vi "Speed Sensitivity.vi"(10 "Joystick \nValue":dbl format="%#_13g") -> (2 "Speed\nOutput":dbl)   [LabVIEW 2014]
panel:
  in  "Shift the\nParabola":dbl
  in  "Full Power\nSetpoint":dbl=0.99 format="%#_13g"
  # "Parabolic Controls"
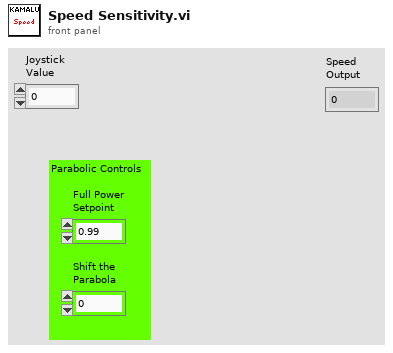
[diagram p1: front panel]
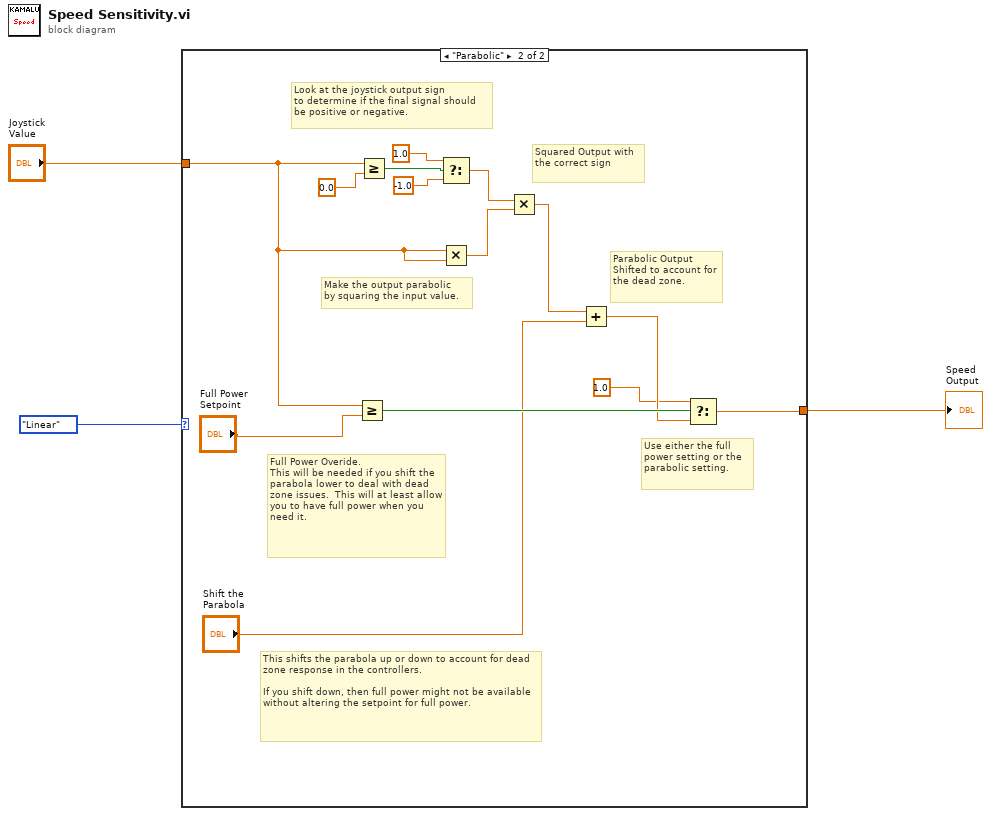
[diagram p0: block diagram]
diagram:
  n1 = case shown="\"Parabolic\"" enum16{"", "Linear", "Parabolic"}."Linear" {
    tunnel: "Joystick \nValue" -> [w4 w14]
    tunnel: [w4 w7] -> w2
    frame "Linear" {
      # "This VI is placed into the Robot Code after the division by 127 has already occured and\nso the input is already the linear mapped output."
    }
    frame "Parabolic" {
      # "Use either the full power setting or the parabolic setting."
      # "This shifts the parabola up or down to account for dead zone response in the controllers.\n\nIf you shift down, then full power might not be available without altering the setpoint for full power."
      # "Parabolic Output\nShifted to account for the dead zone."
      # "Squared Output with the correct sign"
      # "Full Power Overide.\nThis will be needed if you shift the parabola lower to deal with dead zone issues.  This will at least allow you to have full power when you need it."
      # "Make the output parabolic \nby squaring the input value."
      # "Look at the joystick output sign\nto determine if the final signal should\nbe positive or negative."
      n2 = Greater Or Equal?(x=w14, y="Full Power\nSetpoint") -> (x >= y?=w13:bool)
      n3 = Greater Or Equal?(x=w14, y=0.0) -> (x >= y?=w17:bool)
      n4 = Select(t=1.0, s=w17, f=-1.0) -> (s? t:f=w11:dbl)
      n5 = Multiply(x=w14, y=w14) -> (x*y=w12:dbl)
      n6 = Multiply(x=w11, y=w12) -> (x*y=w10:dbl)
      n7 = Add(x=w10, y="Shift the\nParabola") -> (x+y=w9:dbl)
      n8 = Select(t=1.0, s=w13, f=w9) -> (s? t:f=w7:dbl)
    }
  }
  "Speed\nOutput" <- w2
